vi "Temperature Read Hard Mode.vi"() -> ()   [LabVIEW 2020]
panel:
  out "WARNING":bool
  out "Waveform Chart":T1(graph)
  out "START/STOP":bool
  in  "STOP":bool
  in  "START/STOP":bool
  in  "C   or   F":bool
  in  "HIGH Limit":dbl(slide) scale=0.0..100.0
  in  "LOW Limit":dbl(slide) scale=0.0..100.0
  in  "Filename":path
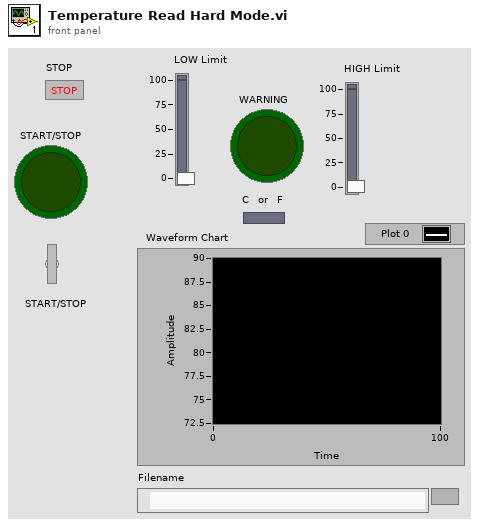
[diagram p1: front panel]
types:
  T1 = cluster{"Temperature (deg F)":dbl, "LOW Limit":dbl, "HIGH Limit":dbl}
  T2 = enum16{"open", "replace", "create", "open or create", "replace or create", "replace or create with confirmation"}
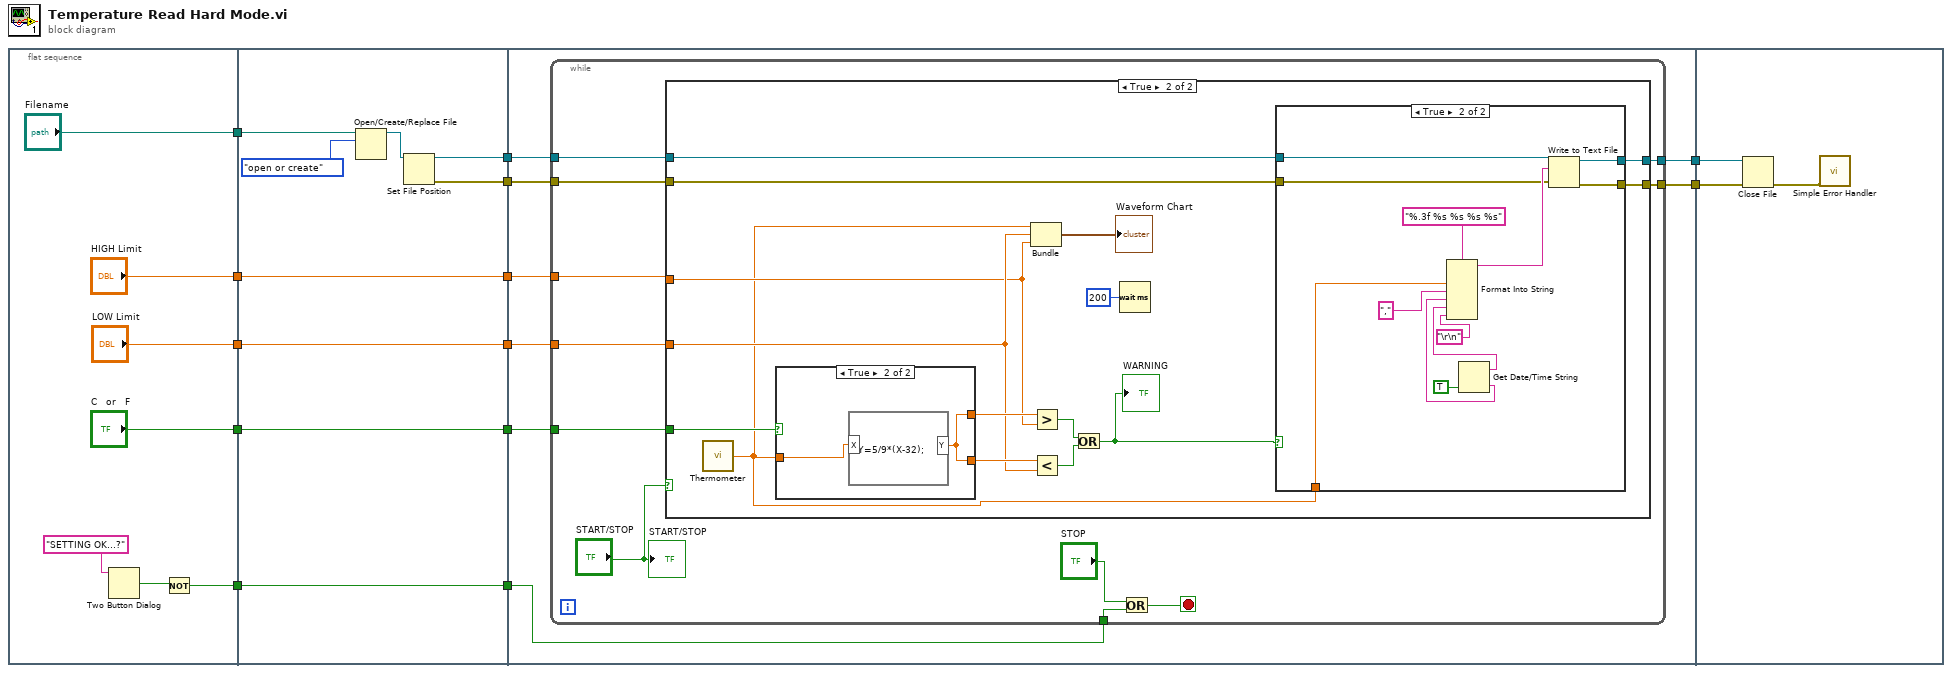
[diagram p0: block diagram]
diagram:
  n1 = flat-sequence {
    tunnel: ["Filename"] -> w13
    tunnel: ["C   or   F"] -> w11
    tunnel: ["LOW Limit"] -> w9
    tunnel: [w15] -> w7
    tunnel: ["HIGH Limit"] -> w1
    tunnel: w13 -> [w29]
    tunnel: [w26] -> w12
    tunnel: w11 -> [w26]
    tunnel: [w25] -> w10
    tunnel: w9 -> [w25]
    tunnel: [w24] -> w8
    tunnel: w7 -> [w24]
    tunnel: [w23] -> w6
    tunnel: [w22] -> w5
    tunnel: [w21] -> w2
    tunnel: w1 -> [w21]
    tunnel: w12 -> [w37]
    tunnel: w10 -> [w36]
    tunnel: w8 -> [w35]
    tunnel: w6 -> [w34]
    tunnel: w5 -> [w33]
    tunnel: [w32] -> w4
    tunnel: [w31] -> w3
    tunnel: w2 -> [w30]
    tunnel: w4 -> [w85]
    tunnel: w3 -> [w84]
    frame #0 {
      n2 = Two Button Dialog(message="SETTING OK...?") -> (T button?=w16:bool)  [unwired: 2 in]
      n3 = Not(x=w16) -> (.not. x?=w15:bool)
    }
    frame #1 {
      n4 = Open/Create/Replace File(file path (use dialog)=w29, operation (0:open)=T2."open or create") -> (refnum out=w27:refnum<file>)  [unwired: 4 in, 2 out]
      n5 = Set File Position(refnum=w27) -> (refnum out=w23:refnum<file>, error out=w22:errorcluster)  [unwired: 3 in]
    }
    frame #2 {
      n6 = while {
        tunnel: w37 -> [w47]
        tunnel: w36 -> [w46]
        tunnel: w35 -> [w43]
        tunnel: w34 -> [w42]
        tunnel: w33 -> [w41]
        tunnel: [w40] -> w32
        tunnel: [w39] -> w31
        tunnel: w30 -> [w38]
        stop <- w44 stop-if-true
        n7 = case shown="True" "START/STOP" {
          tunnel: w47 -> [_ w65]
          tunnel: w38 -> [_ w59]
          tunnel: w46 -> [_ w60]
          tunnel: w42 -> [w50 w54]
          tunnel: w41 -> [w49 w53]
          tunnel: [w50 w52] -> w40
          tunnel: [w49 w51] -> w39
          frame False {
          }
          frame True {
            n8 = call "Thermometer.vi"() -> ("Temperature (deg F)"=w55:dbl)  [unwired: 1 in]
            n9 = case shown="True" w65 {
              tunnel: w55 -> [w80 w82]
              tunnel: [w80 w81] -> w64
              tunnel: [w80 w81] -> w63
              frame False {
              }
              frame True {
                n10 = formula code="Y=5/9*(X-32);"("X"=w82) -> ("Y"=w81:dbl)
              }
            }
            n11 = Bundle("Temperature (deg F)"=w55, "LOW Limit"=w60, "HIGH Limit"=w59) -> (→"Waveform Chart":T1)  [unwired: 1 in]
            n12 = Greater?(x=w64, y=w59) -> (0:w62:bool)
            n13 = Less?(x=w63, y=w60) -> (x < y?=w61:bool)
            n14 = Or(x=w62, y=w61) -> (x .or. y?=w57:bool)
            "WARNING" <- w57
            n15 = Wait (ms)(milliseconds to wait=u32 200) -> ()  [unwired: 1 out]
            n16 = case shown="True" w57 {
              tunnel: w55 -> [_ w77]
              tunnel: w54 -> [w66 w72]
              tunnel: w53 -> [w67 w71]
              tunnel: [w66 w70] -> w52
              tunnel: [w67 w69] -> w51
              frame False {
              }
              frame True {
                n17 = Get Date/Time String(want seconds? (F)=TRUE) -> (date string=w76:string, time string=w75:string)  [unwired: 2 in]
                n18 = Format Into String(format string="%.3f %s %s %s %s", w77, "," ("input 2"), w75, w76, "\r\n") -> (resulting string=w73:string)  [unwired: 2 in, 1 out]
                n19 = Write to Text File(file (use dialog)=w72, text=w73, error in=w71) -> (refnum out=w70:refnum<file>, error out=w69:errorcluster)  [unwired: 1 in, 1 out]
              }
            }
          }
        }
        n20 = Or(x="STOP", y=w43) -> (x .or. y?=w44:bool)
        "START/STOP" <- "START/STOP"
      }
    }
    frame #3 {
      n21 = Close File(refnum=w85, error in=w84) -> (error out=w83:errorcluster)  [unwired: 1 out]
      n22 = call <vilib>:"Simple Error Handler.vi"("error in (no error)"=w83) -> ()  [unwired: 4 in, 5 out]
    }
  }
